vi "Integral_todos.vi"(8 "String Acelerômetro":string, 9 "Última velocidade":dbl, 10 "Última aceleração":dbl, 11 "Último tempo":dbl) -> ()   [LabVIEW 2016]
panel:
  in  "Tempo atual":dbl
  out "Velocidade":dbl
  out "Posição":dbl
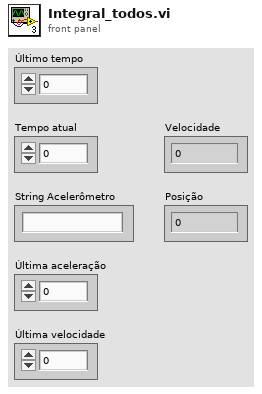
[diagram p1: front panel]
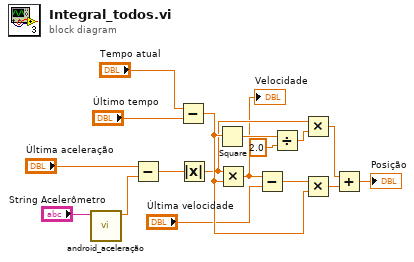
[diagram p0: block diagram]
diagram:
  n1 = call "android_aceleração.vi"("Dados Sensor"="String Acelerômetro") -> ("Aceleração"=w9:dbl)  [unwired: 10 in]
  n2 = Subtract(x="Última aceleração", y=w9) -> (x-y=w8:dbl)
  n3 = Subtract(x="Tempo atual", y="Último tempo") -> (x-y=w15:dbl)
  n4 = Absolute Value(x=w8) -> (abs(x)=w12:dbl)
  n5 = Square(x=w15) -> (x^2=w10:dbl)
  n6 = Multiply(x=w12, y=w15) -> (x*y=w2:dbl)
  "Velocidade" <- w2
  n7 = Subtract(x=w2, y="Última velocidade") -> (x-y=w1:dbl)
  n8 = Divide(x=w10, y=2.0) -> (x/y=w13:dbl)
  n9 = Multiply(x=w12, y=w13) -> (x*y=w14:dbl)
  n10 = Multiply(x=w1, y=w15) -> (x*y=w16:dbl)
  n11 = Add(x=w14, y=w16) -> (x+y=→"Posição":dbl)
